vi "Window template.vi"() -> (3 "Cancelled?":bool)   [LabVIEW 2017]
doc: "Use this template to create a dialog box with event handling."
uses:
  Global Variables/General Globals.vi
panel:
  in  "OK":bool
  # "Section Title"
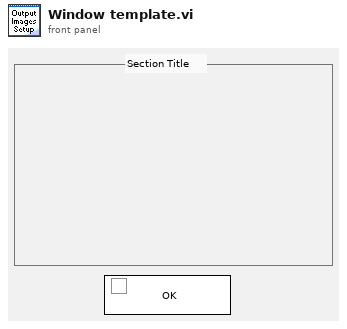
[diagram p1: front panel]
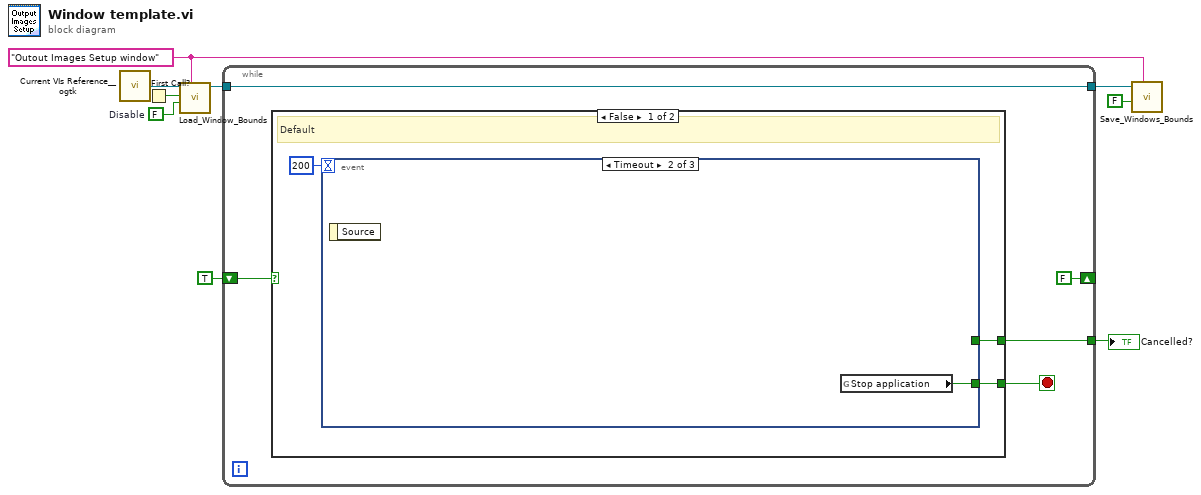
[diagram p0: block diagram]
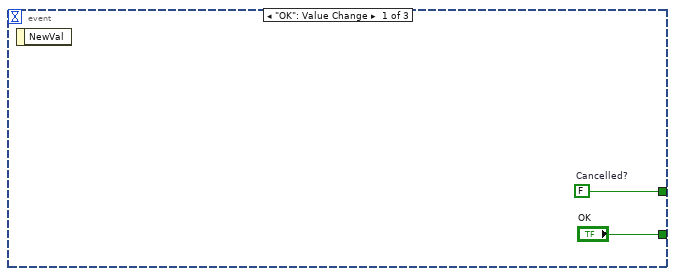
[diagram p2: hidden frame]
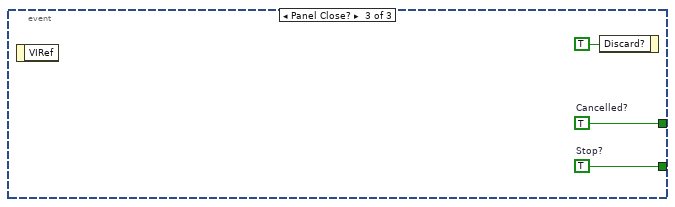
[diagram p3: hidden frame]
diagram:
  w5 = FALSE  # Disable
  w4 = "Outout Images Setup window" ("Window Name (i.e. Key)")
  n1 = call <userlib>:"Current VIs Reference__ogtk.vi"() -> ("Current VI's reference"=w7:refnum<vi>)  [unwired: 5 in]
  n2 = First Call?() -> (First Call?: T/F=w6:bool)
  n3 = call "Load_Window_Bounds.vi"("Window Name (i.e. Key)"=w4, "Disable"=w5, "First Call"=w6, "Window VI's Ref"=w7) -> ("reference out"=w2:refnum<vi>)  [unwired: 4 in, 3 out]
  n4 = while {
    tunnel: [w13] -> w9
    shift-right: [FALSE] -> _
    shift-left: TRUE -> [w12]
    tunnel: w2 -> [w10]
    tunnel: [w10] -> w1
    stop <- w14 stop-if-true
    n5 = case shown="False" w12 {
      tunnel: [w17 _] -> w14
      tunnel: [w16 _] -> w13
      frame False {
        # "Default"
        n6 = event shown="[1] Timeout" {
          selector: _ -> [_ _ _]
          dyn-events: _ -> [_ _ _]
          timeout: 200 -> [_ _ _]
          tunnel: ["OK" w20 w22] -> w17
          tunnel: [w19 _ w21] -> w16
          event "OK": Value Change {
            w19 = FALSE  # Cancelled?
            n7 = event-data() -> ()  [unwired: 1 in, 1 out]
          }
          event Timeout {
            n8 = event-data() -> ()  [unwired: 1 in, 1 out]
            n9 = global read "General Globals.vi" "Stop application"() -> (w20:bool)
          }
          event Panel Close? {
            w21 = TRUE  # Cancelled?
            w22 = TRUE  # Stop?
            n10 = event-data() -> ()  [unwired: 1 in, 1 out]
            n11 = event-data("Discard?"=TRUE) -> ()  [unwired: 1 in, 1 out]
          }
        }
      }
      frame True {
        # "Initialise"
      }
    }
  }
  "Cancelled?" <- w9
  n12 = call "Save_Windows_Bounds.vi"("Window Name (i.e. Key)"=w4, "Front Panel Window:Open"=FALSE, "Window VI's Ref"=w1) -> ()  [unwired: 8 in, 1 out]
